vi "Terminate.vi"(8 "error in (no error)":errorcluster, 10 "Message in":refnum<class "TerminateMessage.lvclass">, 11 "DAQCascade512II in":refnum<class "DAQCascade512II.lvclass">) -> (0 "error out":errorcluster, 3 "DAQCascade512II out":refnum<class "DAQCascade512II.lvclass">)   [LabVIEW 2012, in "DAQCascade512II.lvclass"]
doc: "This member function is called when the statemachine in the run.vi receives an 'terminate' command. It closes the RabbitMQ connection. \n\nOverride this member function in your derived class to release all previously acquired resources (but don't forget to call the parent method). If your component has subcomponents, they count as resources, and you have to release them by calling their own terminate functions."
uses:
  DAQCascade512II.lvclass
  <vilib>/Distrio/Murmex/TerminateMessage/TerminateMessage.lvclass
  <vilib>/Distrio/Murmex/Murmex/Murmex.lvclass
  DAQCascade512II.lvclass/DAQCascade512II.ctl
panel:
  in  "error in":errorcluster
  # "This method is called when the TERMINATE\ntrigger is sent. \n\nOverride this method when your component needs to\nrespond to this trigger. \n\nCall parent for proper implementation"
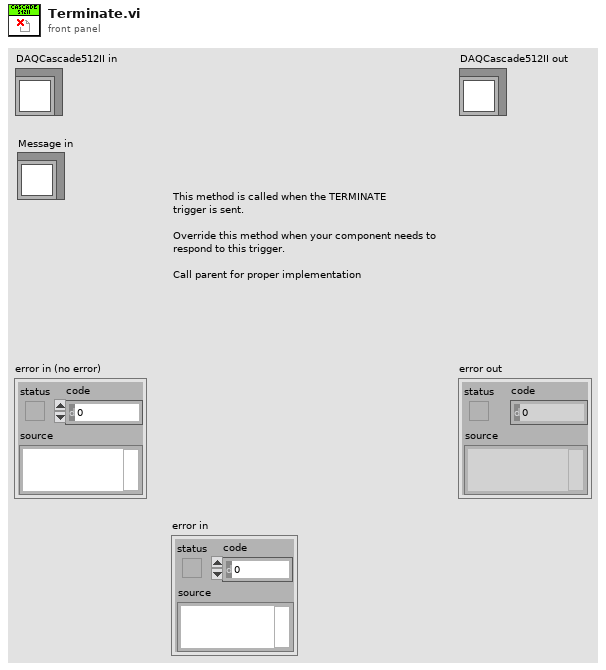
[diagram p1: front panel]
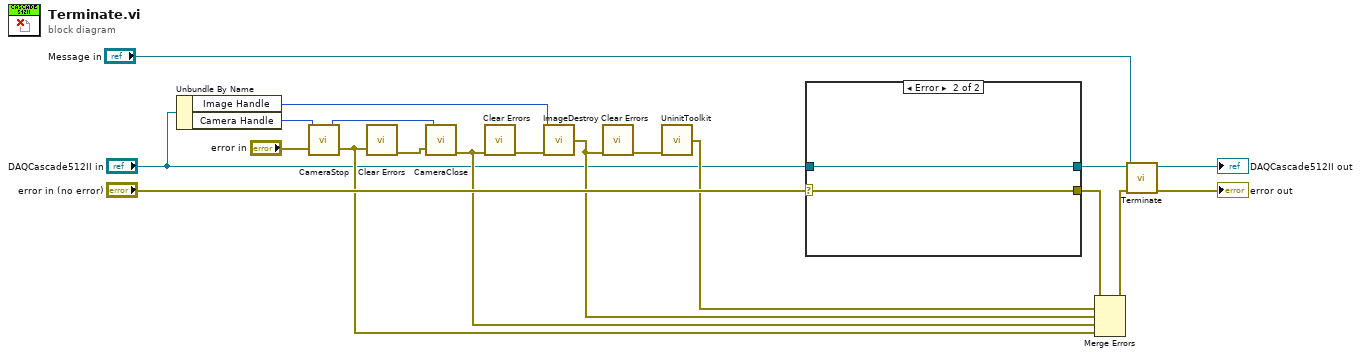
[diagram p0: block diagram]
diagram:
  n1 = Unbundle By Name("DAQCascade512II in") -> ("Image Handle"=w12:u32, "Camera Handle"=w2:u32)
  n2 = call <userlib>:"CameraStop.vi"("error in"="error in", "Camera Handle"=w2) -> ("error out"=w5:errorcluster, "Camera Handle"=w13:u32)
  n3 = call <vilib>:"Clear Errors.vi"("error in (no error)"=w5) -> ("error out"=w16:errorcluster)  [unwired: 6 in]
  n4 = call <userlib>:"CameraClose.vi"("error in"=w16, "Camera Handle"=w13) -> ("error out"=w6:errorcluster)
  n5 = call <vilib>:"Clear Errors.vi"("error in (no error)"=w6) -> ("error out"=w15:errorcluster)  [unwired: 6 in]
  n6 = call <userlib>:"ImageDestroy.vi"("error in"=w15, "Data handle"=w12) -> ("error out"=w7:errorcluster)
  n7 = call <vilib>:"Clear Errors.vi"("error in (no error)"=w7) -> ("error out"=w14:errorcluster)  [unwired: 6 in]
  n8 = call <userlib>:"UninitToolkit.vi"("error in"=w14) -> ("error out"=w8:errorcluster)
  n9 = case shown="Error" "error in (no error)" {
    selector: "error in (no error)" -> [w21 w23]
    tunnel: [w21 w23] -> w4
    tunnel: "DAQCascade512II in" -> [w20 w22]
    tunnel: [w20 w22] -> w9
    frame No Error {
    }
    frame Error {
    }
  }
  n10 = Merge Errors(w4, w8, w7, w6, w5) -> (w1:errorcluster)
  n11 = call-parent "Terminate.vi"("error in (no error)"=w1, "Message in"="Message in", "Murmex in"=w9) -> ("error out"=→"error out":errorcluster, "Murmex out"=→"DAQCascade512II out":refnum<class "DAQCascade512II.lvclass">)  [unwired: 7 in]
